vi "Version 1_Read Batch Setpoint.vi"(7 "Unit ID (A)":string="A", 8 "error in":errorcluster, 10 "Legacy Status (optional - wire for speed)":u8(ring) items=["Rev. 21 Board", "Rev. 22 Board", "Rev. 23 Board"], 11 "VISA Session In":refnum<visa-resource-name>="Alicat") -> (0 "error out":errorcluster, 1 "Register 92 Value (DBL)":dbl, 3 "VISA Session Out":refnum<visa-resource-name>)   [LabVIEW 2015]
doc: "Reads the value of the register containing the batch setpoint value in the Alicat device. ONLY AVAILABLE FOR R22 BOARDS (run \"Legacy Detector\" to determine board revision). Does nothing if the device is not a controller with the totalizer activated and a firmware version greater than 4v33 (run \"Batch detect\" to determine whether a unit has batching available)."
uses:
  <vilib>/Instr/_visa.llb/VISA Flush IO Buffer Mask.ctl
panel:
  # "ONLY AVAILABLE FOR R22 BOARDS AND ABOVE\n(provided it is a controller with totalizer and at least firmware 4v33)"
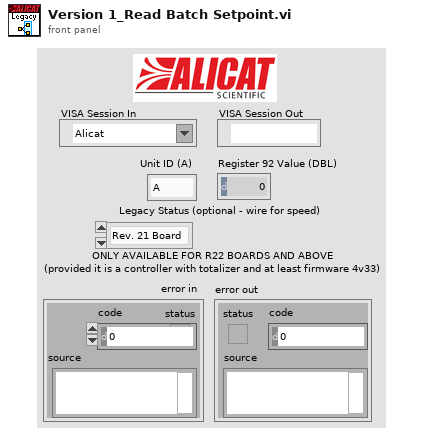
[diagram p1: front panel]
types:
  T1 = typedef "VISA Flush IO Buffer Mask.ctl" = u16
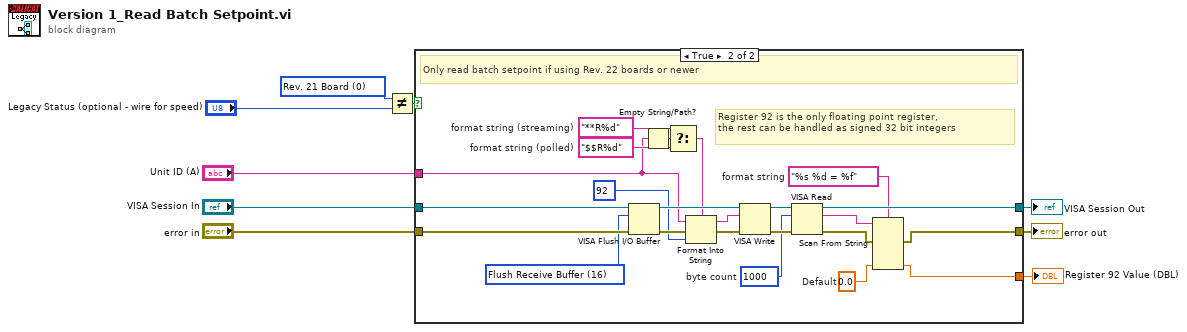
[diagram p0: block diagram]
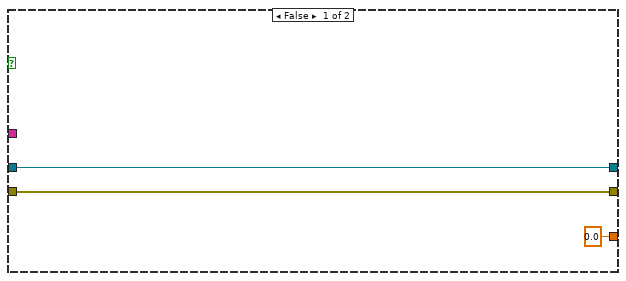
[diagram p2: hidden frame]
diagram:
  w2 = u8 0 items=["Rev. 21 Board", "Rev. 22 Board", "Rev. 23 Board"] ("Legacy Status")
  n1 = Not Equal?(x=w2, y="Legacy Status (optional - wire for speed)") -> (x != y?=w3:bool)
  n2 = case shown="True" w3 {
    tunnel: "VISA Session In" -> [w12 w34]
    tunnel: "error in" -> [w11 w32]
    tunnel: [w11 w28] -> w7
    tunnel: [w12 w27] -> w6
    tunnel: "Unit ID (A)" -> [_ w15]
    tunnel: [0.0 ("Default") w13] -> w4
    frame False {
    }
    frame True {
      w16 = "**R%d"  # format string (streaming)
      w20 = 0.0  # Default
      w18 = "$$R%d"  # format string (polled)
      w31 = T1 16 items=["Flush Receive Buffer"=16, "Write Transmit Buffer to Device"=32, "Flush Receive Buffer (No I/O)"=64, "Flush Transmit Buffer"=128] ("Mask")
      w24 = "%s %d = %f"  # format string
      w25 = u32 1000  # byte count
      # "Register 92 is the only floating point register, \nthe rest can be handled as signed 32 bit integers"
      # "Only read batch setpoint if using Rev. 22 boards or newer"
      n3 = VISA Flush I/O Buffer(VISA resource name=w34, mask (16)=w31, error in (no error)=w32) -> (VISA resource name out=w33:refnum<visa-resource-name>, error out=w22:errorcluster)
      n4 = Empty String/Path?(string/path=w15) -> (empty?=w17:bool)
      n5 = Select(t=w16, s=w17, f=w18) -> (s? t:f=w14:string)
      n6 = Format Into String(format string=w14, initial string=w15, error in=w22, u16 92 ("Register address")) -> (resulting string=w23:string, error out=w21:errorcluster)
      n7 = VISA Write(VISA resource name=w33, write buffer=w23, error in (no error)=w21) -> (VISA resource name out=w30:refnum<visa-resource-name>, error out=w35:errorcluster)  [unwired: 1 out]
      n8 = VISA Read(VISA resource name=w30, byte count=w25, error in (no error)=w35) -> (VISA resource name out=w27:refnum<visa-resource-name>, read buffer=w26:string, error out=w29:errorcluster)  [unwired: 1 out]
      n9 = Scan From String(format string=w24, input string=w26, error in=w29, default 3=w20) -> (error out=w28:errorcluster, output 3=w13:dbl)  [unwired: 5 in, 2 out]
    }
  }
  "error out" <- w7
  "VISA Session Out" <- w6
  "Register 92 Value (DBL)" <- w4
